vi "FGV_PCO_Timings.vi"(3 "error in":errorcluster, 4 "Timings (sleep, expo, readout) _s":dbl[](array[numeric])=[0.025, 0.1, 0.02], 5 "Action":T1) -> (0 "error out":errorcluster, 1 "Timings (sleep, expo, readout) _s":dbl[](array[numeric])=[0.025, 0.1, 0.02])   [LabVIEW 2026]
uses:
  Controls/TypeDef_FGV.ctl
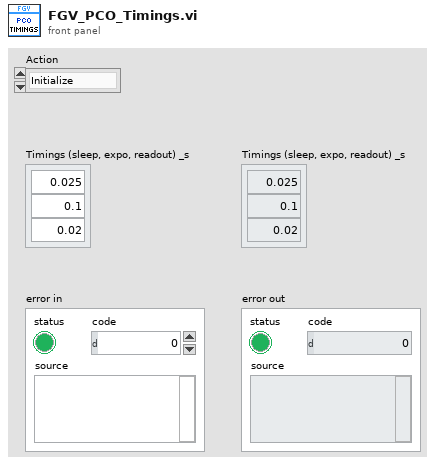
[diagram p1: front panel]
types:
  T1 = typedef "TypeDef_FGV.ctl" = enum16{"Initialize", "Write", "Read"}
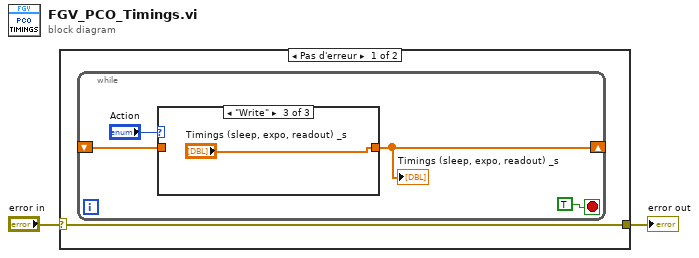
[diagram p0: block diagram]
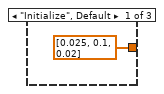
[diagram p2: hidden frame]
diagram:
  n1 = case shown="Pas d'erreur" "error in" {
    selector: "error in" -> [w3 w11]
    tunnel: [w3 w11] -> w2
    frame No Error {
      n2 = while {
        shift-right: [w4] -> _
        shift-left: _ -> [w5]
        stop <- TRUE stop-if-true
        n3 = case shown="\"Write\"" "Action" {
          tunnel: [dbl[] [0.025, 0.1, 0.02] ("Timings (sleep, expo, readout) _s") w9 "Timings (sleep, expo, readout) _s"] -> w4
          tunnel: w5 -> [_ w9 _]
          frame "Initialize", Default {
          }
          frame "Read" {
          }
          frame "Write" {
          }
        }
        "Timings (sleep, expo, readout) _s" <- w4
      }
    }
    frame Error {
    }
  }
  "error out" <- w2
